vi "MHM Load Register.vi"(6 "pulNumerOfBytes":u32, 8 "error in (no error)":errorcluster, 9 "ulAdr":u32, 10 "pcFilename":string, 11 "ulMHMHandle":u32) -> (0 "error out":errorcluster, 1 "pulNumberOfBytes out":u32, 2 "pulData":u32[](array[numeric]), 3 "function return":u32)   [LabVIEW 2019, in "MHM_1SL_interface.lvlib"]
uses:
  MHM_1SL_interface.lvlib
  lib/MHM_1SL_interface.dll
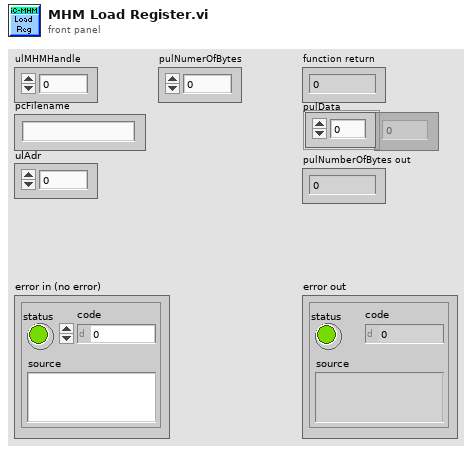
[diagram p1: front panel]
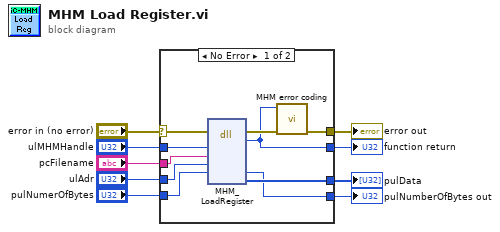
[diagram p0: block diagram]
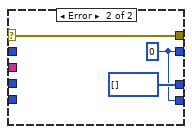
[diagram p2: hidden frame]
diagram:
  n1 = case shown="No Error" "error in (no error)" {
    selector: "error in (no error)" -> [w19 w22]
    tunnel: "ulMHMHandle" -> [w18 _]
    tunnel: [w16 w22] -> w8
    tunnel: [w15 w20] -> w9
    tunnel: "pcFilename" -> [w14 _]
    tunnel: "ulAdr" -> [w13 _]
    tunnel: "pulNumerOfBytes" -> [w12 _]
    tunnel: [w11 u32[] [] ("pulData")] -> w2
    tunnel: [w10 w20] -> w1
    frame No Error {
      n2 = dll-call lib="C:/workspace/project/scancon/MHM_1SL_interface_4.4.0/lv_interface/lib/MHM_1SL_interface.dll" fn="MHM_LoadRegister"(error in=w19, "ulMHMHandle"=w18, "pcFilename"=w14, "ulAdr"=w13, "pulNumerOfBytes"=w12) -> (error out=w17:errorcluster, "return type"=w15:u32, "pulNumerOfBytes"=w10:u32, "pulData"=w11:u32[])  [unwired: 6 in, 1 out]
      n3 = call "MHM error coding.vi"("error in (no error)"=w17, "function return in"=w15) -> ("error out"=w16:errorcluster)  [unwired: 9 in]
    }
    frame Error {
      w20 = u32 0 ("return type")
    }
  }
  "function return" <- w9
  "error out" <- w8
  "pulData" <- w2
  "pulNumberOfBytes out" <- w1
